vi "tb_twiddle factor generation.vi"() -> ()   [LabVIEW 2011]
uses:
  <vilib>/measure/NI_MAPro.lvlib
  <vilib>/measure/maspectr.llb/FFT Spectrum (Mag-Phase) for 1 Chan.vi
panel:
  out "Output Valid":bool[](array[boolean])
  out "FXP Twiddle":cdb[](array[numeric])
  out "Error Spectrum":cluster{"f0":dbl, "df":dbl, "magnitude":dbl[]}(graph)
  out "Error Signal":dbl[](graph)
  out "FLP LV phase":dbl[](array[numeric])
  out "Floating Point Twiddle (LV)":cdb[](array[numeric])
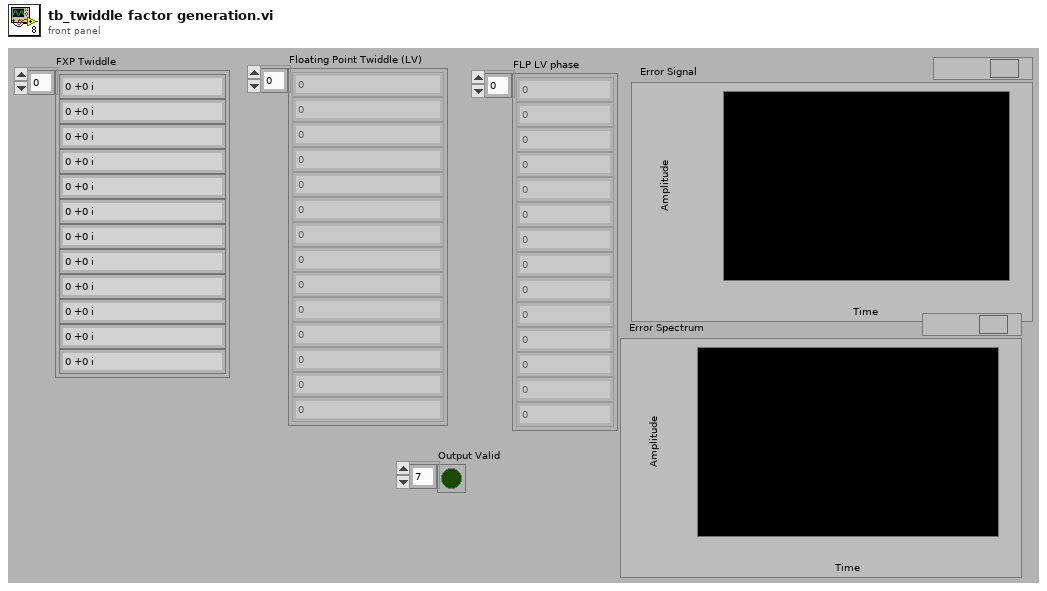
[diagram p1: front panel]
types:
  T1 = cluster{"dB On (F)":bool, "unwrap phase (F)":bool, "convert to degree (F)":bool}
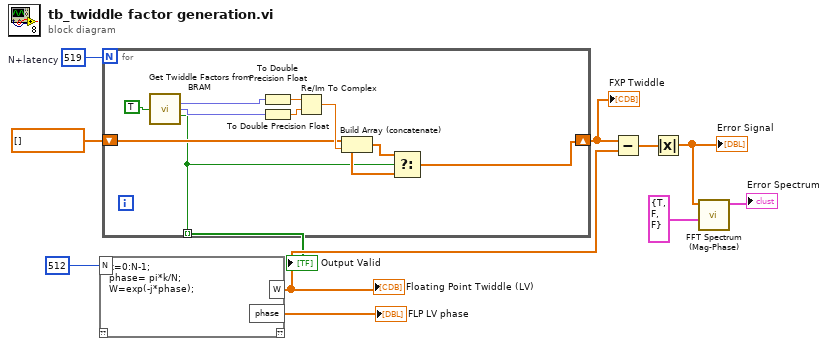
[diagram p0: block diagram]
diagram:
  w11 = 519  # N+latency
  n1 = mathscript code="k=0:N-1;\nphase= pi*k/N;\nW=exp(-j*phase);"("N"=512) -> ("W"=w8:cdb[], "phase"=→"FLP LV phase":dbl[])  [unwired: 1 in, 1 out]
  "Floating Point Twiddle (LV)" <- w8
  n2 = for {
    N: w11 -> [_]
    shift-right: [w13] -> w2
    shift-left: cdb[] [] -> [w14]
    tunnel: [w12] -> w1 mode=indexing
    n3 = call <userlib>:"Get Twiddle Factors from BRAM.vi"("Input Data Valid"=TRUE) -> ("cosine"=w18:fxp<+/-,18,1>, "sine"=w17:fxp<+/-,18,1>, "Output Valid"=w12:bool)  [unwired: 11 in, 1 out]
    n4 = To Double Precision Float(number=w18) -> (double precision float=w19:dbl)
    n5 = To Double Precision Float(number=w17) -> (double precision float=w20:dbl)
    n6 = Re/Im To Complex(1:w20, 2:w19) -> (0:w16:cdb)
    n7 = Build Array (concatenate)(w14, w16) -> (w15:cdb[])
    n8 = Select(t=w15, s=w12, f=w14) -> (s? t:f=w13:cdb[])
  }
  "FXP Twiddle" <- w2
  "Output Valid" <- w1
  n9 = Subtract(x=w2, y=w8) -> (x-y=w7:cdb[])
  n10 = Absolute Value(x=w7) -> (abs(x)=w6:dbl[])
  "Error Signal" <- w6
  n11 = call-poly <vilib>:"FFT Spectrum (Mag-Phase).vi"("view"=T1 {"dB On (F)"=TRUE, "unwrap phase (F)"=FALSE, "convert to degree (F)"=FALSE}, "time signal"=w6) -> ("magnitude"=→"Error Spectrum":cluster{"f0":dbl, "df":dbl, "magnitude":dbl[]})  [unwired: 5 in, 4 out]
